vi "disableList.vi"(8 "error in (no error)":errorcluster, 11 "Subnet in":refnum<class "Subnet.lvclass">) -> (0 "error out":errorcluster, 3 "Subnet out":refnum<class "Subnet.lvclass">)   [LabVIEW 2016, in "Subnet.lvclass"]
uses:
  Subnet.lvclass
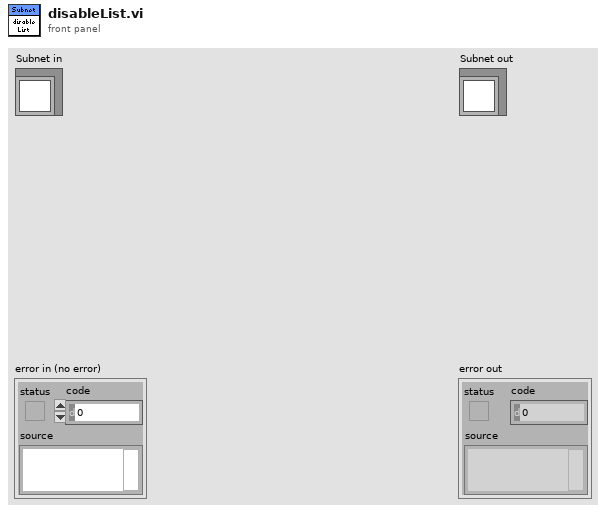
[diagram p1: front panel]
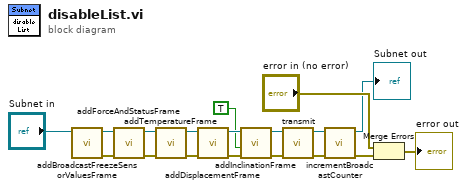
[diagram p0: block diagram]
diagram:
  n1 = call "addBroadcastFreezeSensorValuesFrame.vi"("Subnet in"="Subnet in") -> ("error out"=w10:errorcluster, "Subnet out"=w11:refnum<class "Subnet.lvclass">)  [unwired: 9 in]
  n2 = call "addForceAndStatusFrame.vi"("error in (no error)"=w10, "Subnet in"=w11) -> ("error out"=w5:errorcluster, "Subnet out"=w9:refnum<class "Subnet.lvclass">)  [unwired: 8 in]
  n3 = call "addTemperatureFrame.vi"("error in (no error)"=w5, "Subnet in"=w9) -> ("error out"=w4:errorcluster, "Subnet out"=w8:refnum<class "Subnet.lvclass">)  [unwired: 8 in]
  n4 = call "addDisplacementFrame.vi"("error in (no error)"=w4, "Subnet in"=w8) -> ("error out"=w3:errorcluster, "Subnet out"=w7:refnum<class "Subnet.lvclass">)  [unwired: 8 in]
  n5 = call "addInclinationFrame.vi"("error in (no error)"=w3, "TriggerIRQ"=TRUE, "Subnet in"=w7) -> ("error out"=w2:errorcluster, "Subnet out"=w6:refnum<class "Subnet.lvclass">)  [unwired: 7 in]
  n6 = call "transmit.vi"("error in (no error)"=w2, "Subnet in"=w6) -> ("error out"=w14:errorcluster, "Subnet out"=w16:refnum<class "Subnet.lvclass">)  [unwired: 8 in]
  n7 = call "incrementBroadcastCounter.vi"("error in (no error)"=w14, "Subnet in"=w16) -> ("error out"=w13:errorcluster, "Subnet out"=→"Subnet out":refnum<class "Subnet.lvclass">)  [unwired: 8 in]
  n8 = Merge Errors("error in (no error)", w13) -> (→"error out":errorcluster)
